vi "IPS Get Status.vi"(11 "Return String from Device (Not all commands return a String)":string="X42A1C2H5M12P21\r") -> (0 "System":string="Warming up/On Negative V Limit", 1 "SHeater":string="Heater Fault", 2 "Mode":string="T/Fast/Sweep Limiting", 3 "Activity":string="To Set Point")   [LabVIEW 2013]
panel:
  out "System":string="42"
  out "Mode":string="12"
  out "Activity":dbl=1.0
  out "SHeater":dbl=5.0
  out "System":string="X42"
  out "Activity":string="A1"
  out "LOC/REM":string="C2"
  out "SHeater":string="H5"
  out "Mode":string="M12"
  out "Polarity":string="P21\r"
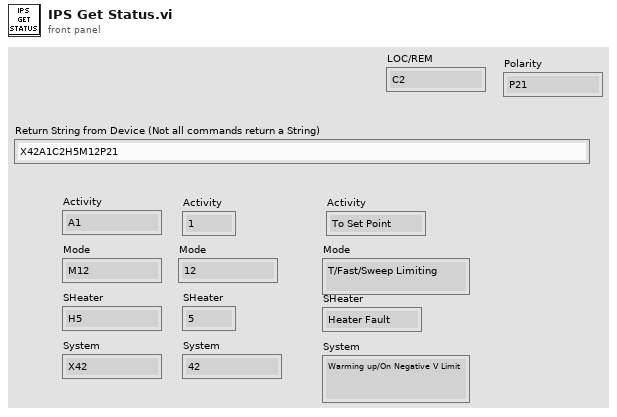
[diagram p1: front panel]
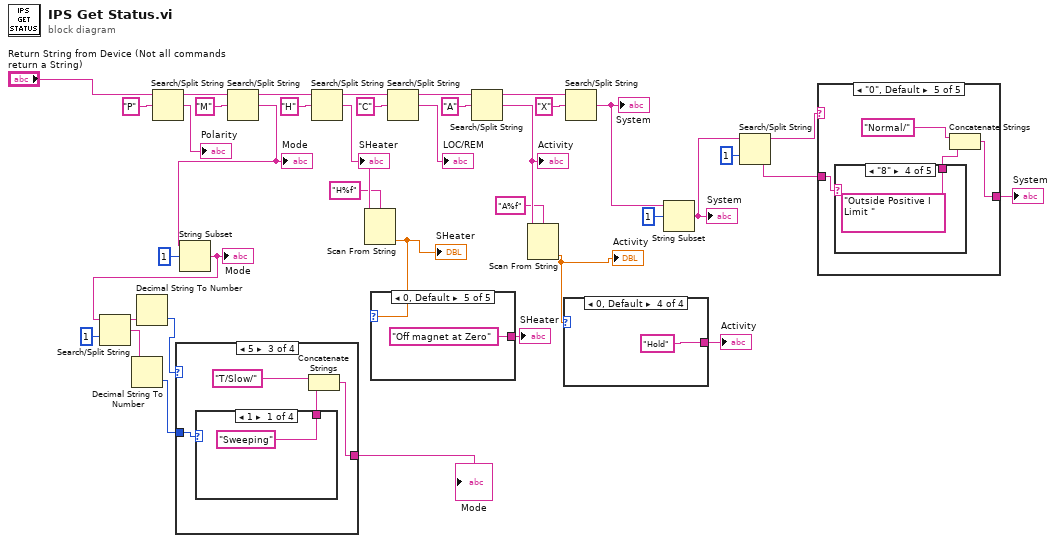
[diagram p0: block diagram]
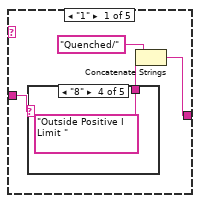
[diagram p2: hidden frame]
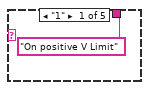
[diagram p3: hidden frame]
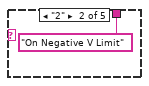
[diagram p4: hidden frame]
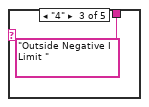
[diagram p5: hidden frame]
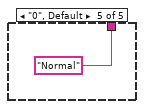
[diagram p6: hidden frame]
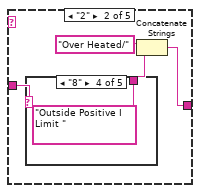
[diagram p7: hidden frame]
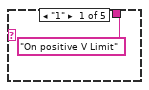
[diagram p8: hidden frame]
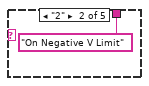
[diagram p9: hidden frame]
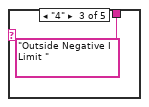
[diagram p10: hidden frame]
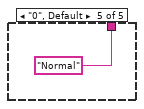
[diagram p11: hidden frame]
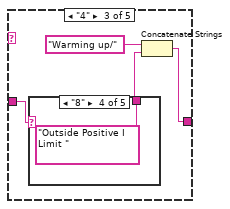
[diagram p12: hidden frame]
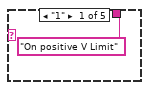
[diagram p13: hidden frame]
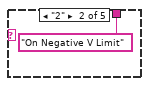
[diagram p14: hidden frame]
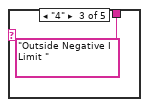
[diagram p15: hidden frame]
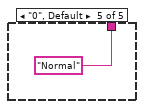
[diagram p16: hidden frame]
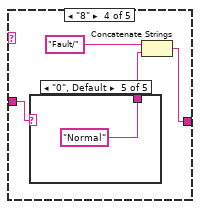
[diagram p17: hidden frame]
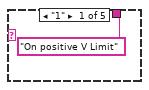
[diagram p18: hidden frame]
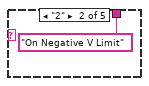
[diagram p19: hidden frame]
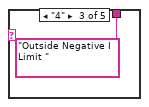
[diagram p20: hidden frame]
diagram:
  n1 = Search/Split String(string="Return String from Device (Not all commands return a String)", search string/char (-)="P") -> (substring before match=w35:string, match + rest of string=→"Polarity":string)  [unwired: 1 in, 1 out]
  n2 = Search/Split String(string=w35, search string/char (-)="M") -> (substring before match=w34:string, match + rest of string=w20:string)  [unwired: 1 in, 1 out]
  "Mode" <- w20
  n3 = String Subset(string=w20, offset (0)=1) -> (substring=w11:string)  [unwired: 1 in]
  "Mode" <- w11
  n4 = Search/Split String(string=w11, offset (0)=1) -> (substring before match=w10:string, match + rest of string=w8:string)  [unwired: 1 in, 1 out]
  n5 = Decimal String To Number(string=w8) -> (number=w7:i32)  [unwired: 2 in, 1 out]
  n6 = Decimal String To Number(string=w10) -> (number=w9:i32)  [unwired: 2 in, 1 out]
  n7 = case shown="5" w9 {
    tunnel: w7 -> [w42 w50 w58 w66]
    tunnel: [w39 w47 w55 w63] -> w6
    frame 1 {
      n8 = case shown="0, Default" w42 {
        tunnel: ["Sweeping" "Sweep Limiting" "Sweeping&Sweep Limiting" "Rest"] -> w40
        frame 1 {
        }
        frame 2 {
        }
        frame 3 {
        }
        frame 0, Default {
        }
      }
      n9 = Concatenate Strings("T/Fast/", w40) -> (w39:string)
    }
    frame 4 {
      n10 = case shown="0, Default" w50 {
        tunnel: ["Sweeping" "Sweep Limiting" "Sweeping&Sweep Limiting" "Rest"] -> w48
        frame 1 {
        }
        frame 2 {
        }
        frame 3 {
        }
        frame 0, Default {
        }
      }
      n11 = Concatenate Strings("A/Slow/", w48) -> (w47:string)
    }
    frame 5 {
      n12 = case shown="1" w58 {
        tunnel: ["Sweeping" "Sweep Limiting" "Sweeping&Sweep Limiting" "Rest"] -> w56
        frame 1 {
        }
        frame 2 {
        }
        frame 3 {
        }
        frame 0, Default {
        }
      }
      n13 = Concatenate Strings("T/Slow/", w56) -> (w55:string)
    }
    frame 0, Default {
      n14 = case shown="3" w66 {
        tunnel: ["Sweeping" "Sweep Limiting" "Sweeping&Sweep Limiting" "Rest"] -> w64
        frame 1 {
        }
        frame 2 {
        }
        frame 3 {
        }
        frame 0, Default {
        }
      }
      n15 = Concatenate Strings("A/Fast/", w64) -> (w63:string)
    }
  }
  "Mode" <- w6
  n16 = Search/Split String(string=w34, search string/char (-)="H") -> (substring before match=w32:string, match + rest of string=w24:string)  [unwired: 1 in, 1 out]
  "SHeater" <- w24
  n17 = Scan From String(format string="H%f", input string=w24) -> (output 1=w16:dbl)  [unwired: 3 in, 3 out]
  "SHeater" <- w16
  n18 = case shown="0, Default" w16 {
    tunnel: ["On" "Off magnet at Field" "Heater Fault" "No Switch Fitted" "Off magnet at Zero"] -> w15
    frame 1 {
    }
    frame 2 {
    }
    frame 5 {
    }
    frame 8 {
    }
    frame 0, Default {
    }
  }
  "SHeater" <- w15
  n19 = Search/Split String(string=w32, search string/char (-)="C") -> (substring before match=w30:string, match + rest of string=→"LOC/REM":string)  [unwired: 1 in, 1 out]
  n20 = Search/Split String(string=w30, search string/char (-)="A") -> (substring before match=w27:string, match + rest of string=w22:string)  [unwired: 1 in, 1 out]
  "Activity" <- w22
  n21 = Scan From String(format string="A%f", input string=w22) -> (output 1=w14:dbl)  [unwired: 3 in, 3 out]
  "Activity" <- w14
  n22 = case shown="0, Default" w14 {
    tunnel: ["To Set Point" "To Zero" "Clamped" "Hold"] -> w13
    frame 1 {
    }
    frame 2 {
    }
    frame 4 {
    }
    frame 0, Default {
    }
  }
  "Activity" <- w13
  n23 = Search/Split String(string=w27, search string/char (-)="X") -> (match + rest of string=w17:string)  [unwired: 1 in, 2 out]
  "System" <- w17
  n24 = String Subset(string=w17, offset (0)=1) -> (substring=w4:string)  [unwired: 1 in]
  "System" <- w4
  n25 = Search/Split String(string=w4, offset (0)=1) -> (substring before match=w3:string, match + rest of string=w2:string)  [unwired: 1 in, 1 out]
  n26 = case shown="\"0\", Default" w3 {
    tunnel: [w82 w91 w100 w109 w117] -> w1
    tunnel: w2 -> [w80 w89 w98 w107 w116]
    frame "1" {
      n27 = case shown="\"8\"" w80 {
        tunnel: ["On positive V Limit" "On Negative V Limit" "Outside Negative I Limit " "Outside Positive I Limit " "Normal"] -> w81
        frame "1" {
        }
        frame "2" {
        }
        frame "4" {
        }
        frame "8" {
        }
        frame "0", Default {
        }
      }
      n28 = Concatenate Strings("Quenched/", w81) -> (w82:string)
    }
    frame "2" {
      n29 = case shown="\"8\"" w89 {
        tunnel: ["On positive V Limit" "On Negative V Limit" "Outside Negative I Limit " "Outside Positive I Limit " "Normal"] -> w90
        frame "1" {
        }
        frame "2" {
        }
        frame "4" {
        }
        frame "8" {
        }
        frame "0", Default {
        }
      }
      n30 = Concatenate Strings("Over Heated/", w90) -> (w91:string)
    }
    frame "4" {
      n31 = case shown="\"8\"" w98 {
        tunnel: ["On positive V Limit" "On Negative V Limit" "Outside Negative I Limit " "Outside Positive I Limit " "Normal"] -> w99
        frame "1" {
        }
        frame "2" {
        }
        frame "4" {
        }
        frame "8" {
        }
        frame "0", Default {
        }
      }
      n32 = Concatenate Strings("Warming up/", w99) -> (w100:string)
    }
    frame "8" {
      n33 = case shown="\"0\", Default" w107 {
        tunnel: ["On positive V Limit" "On Negative V Limit" "Outside Negative I Limit " "Outside Positive I Limit " "Normal"] -> w108
        frame "1" {
        }
        frame "2" {
        }
        frame "4" {
        }
        frame "8" {
        }
        frame "0", Default {
        }
      }
      n34 = Concatenate Strings("Fault/", w108) -> (w109:string)
    }
    frame "0", Default {
      n35 = case shown="\"8\"" w116 {
        tunnel: ["On positive V Limit" "On Negative V Limit" "Outside Negative I Limit " "Outside Positive I Limit " "Normal"] -> w118
        frame "1" {
        }
        frame "2" {
        }
        frame "4" {
        }
        frame "8" {
        }
        frame "0", Default {
        }
      }
      n36 = Concatenate Strings("Normal/", w118) -> (w117:string)
    }
  }
  "System" <- w1
